vi "AlliGator Get Local Fit Results String.vi"(6 "Decay Sum":dbl, 8 "Parameters":dbl[](array[numeric]), 9 "Y":i32, 10 "X":i32, 11 "[Decay Fit Parameter Name]":T1[](array[typedef])) -> (3 "Fit Results String":string)   [LabVIEW 2021, in "AlliGator Decay Fit Parameter Map.lvlib"]
doc: "Builds Decay Fit Parmeters string."
uses:
  AlliGator Decay Fit Parameter Map.lvlib
  Fits/IRF(X)PSED/Decay Fit Parameters & Derived Quantities List.ctl
  Fits/Fits.lvlib
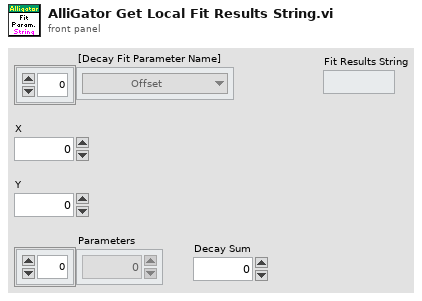
[diagram p1: front panel]
types:
  T1 = typedef "Fits.lvlib/Decay Fit Parameters & Derived Quantities List.ctl" = enum16{"Offset", "Baseline", "A_1", "tau_1", "A_2", "tau_2", "<tau>_a", "f1_a", "f2_a", "<tau>_i", "f1_i", "f2_i", "-", "R^2", "Chi^2"}
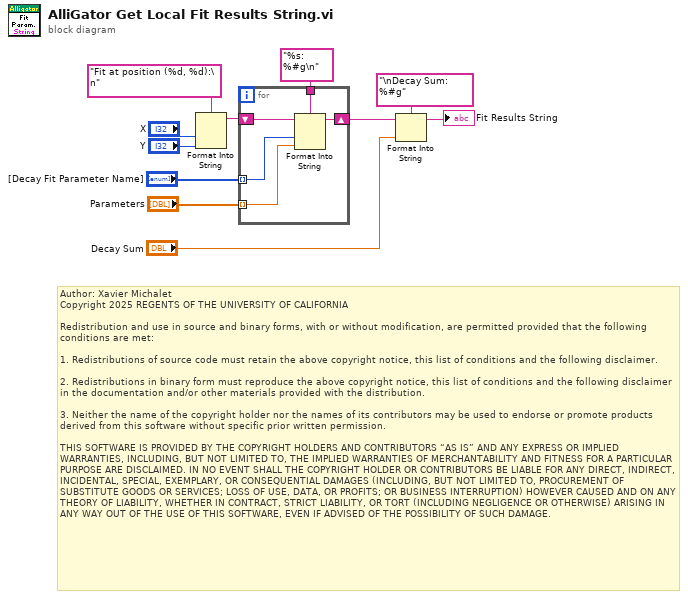
[diagram p0: block diagram]
diagram:
  # "Author: Xavier Michalet\nCopyright 2025 REGENTS OF THE UNIVERSITY OF CALIFORNIA\n\nRedistribution and use in source and binary forms, with or without modification, are permitted provided that the following conditions are met:\n\n1. Redistributions of source code must retain the above copyright notice, this list of conditions and the following disclaimer.\n\n2. Redistributions in binary form must reproduce the above copyright notice, this list of conditions and the following disclaimer in the documentation and/or other materials provided with the distribution.\n\n3. Neither the name of the copyright holder nor the names of its contributors may be used to endorse or promote products derived from this software without specific prior written permission.\n\nTHIS SOFTWARE IS PROVIDED BY THE COPYRIGHT HOLDERS AND CONTRIBUTORS “AS IS” AND ANY EXPRESS OR IMPLIED WARRANTIES, INCLUDING, BUT NOT LIMITED TO, THE IMPLIED WARRANTIES OF MERCHANTABILITY AND FITNESS FOR A PARTICULAR PURPOSE ARE DISCLAIMED. IN NO EVENT SHALL THE COPYRIGHT HOLDER OR CONTRIBUTORS BE LIABLE FOR ANY DIRECT, INDIRECT, INCIDENTAL, SPECIAL, EXEMPLARY, OR CONSEQUENTIAL DAMAGES (INCLUDING, BUT NOT LIMITED TO, PROCUREMENT OF SUBSTITUTE GOODS OR SERVICES; LOSS OF USE, DATA, OR PROFITS; OR BUSINESS INTERRUPTION) HOWEVER CAUSED AND ON ANY THEORY OF LIABILITY, WHETHER IN CONTRACT, STRICT LIABILITY, OR TORT (INCLUDING NEGLIGENCE OR OTHERWISE) ARISING IN ANY WAY OUT OF THE USE OF THIS SOFTWARE, EVEN IF ADVISED OF THE POSSIBILITY OF SUCH DAMAGE."
  n1 = Format Into String(format string="Fit at position (%d, %d):\n", "X", "Y") -> (resulting string=w8:string)  [unwired: 2 in, 1 out]
  n2 = for {
    shift-right: [w15] -> w4
    shift-left: w8 -> [w16]
    tunnel: "[Decay Fit Parameter Name]" -> [w14] mode=indexing
    tunnel: "Parameters" -> [w13] mode=indexing
    tunnel: "%s: %#g\n" ("format string") -> [w12]
    n3 = Format Into String(format string=w12, initial string=w16, w14, w13) -> (resulting string=w15:string)  [unwired: 1 in, 1 out]
  }
  n4 = Format Into String(format string="\nDecay Sum: %#g", initial string=w4, "Decay Sum") -> (resulting string=→"Fit Results String":string)  [unwired: 1 in, 1 out]
